vi "Publisher Do.vi"(8 "error in (no error)":errorcluster, 10 "Publisher in":refnum<class "Publisher.lvclass">, 11 "Subscribe Msg":refnum<class "Bypass Msg.lvclass">) -> (0 "error out":errorcluster, 2 "Publisher out":refnum<class "Publisher.lvclass">)   [LabVIEW 2020, in "Publisher.lvlib" / "Bypass Msg.lvclass"]
doc: "The message is dropped by calling the parent method. The Bypass Msg should never end up on the Publisher."
uses:
  Bypass Msg.lvclass
  Publisher/Publisher.lvclass
  Sender Msg/Sender Msg.lvclass
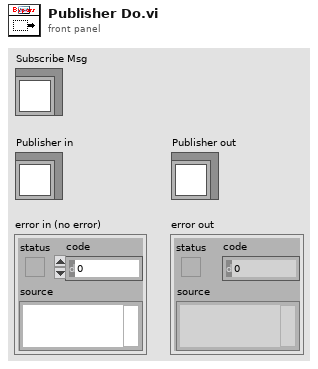
[diagram p1: front panel]
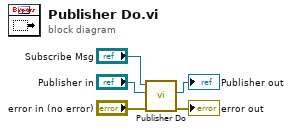
[diagram p0: block diagram]
diagram:
  n1 = call-parent "Publisher Do.vi"("error in (no error)"="error in (no error)", "Publisher in"="Publisher in", "Subscribe Msg"="Subscribe Msg") -> ("error out"=→"error out":errorcluster, "Publisher out"=→"Publisher out":refnum<class "Publisher.lvclass">)  [unwired: 7 in]
